vi "ClusterEscala.vi"() -> ()   [LabVIEW 2020]
panel:
  out "Cluster":T1 {"PRESION" scale=0.0..10.0; "FLUJO" scale=0.0..10.0; "TEMPERATURA" scale=0.0..100.0}
  in  "Cluster 2":T2
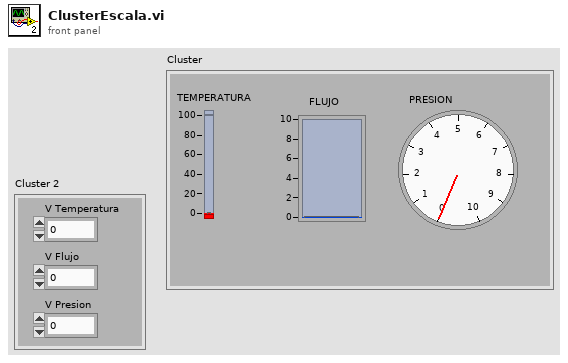
[diagram p1: front panel]
types:
  T1 = cluster{"TEMPERATURA":dbl, "FLUJO":dbl, "PRESION":dbl}
  T2 = cluster{"V Temperatura":dbl, "V Flujo ":dbl, "V Presion ":dbl}
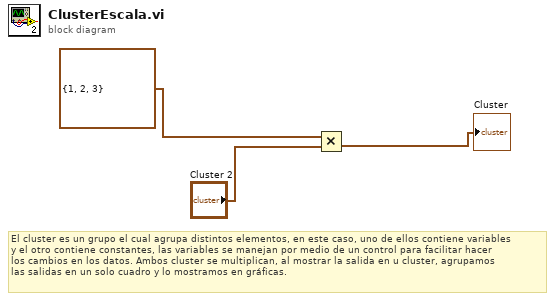
[diagram p0: block diagram]
diagram:
  # "El cluster es un grupo el cual agrupa distintos elementos, en este caso, uno de ellos contiene variables\ny el otro contiene constantes, las variables se manejan por medio de un control para facilitar hacer\nlos cambios en los datos. Ambos cluster se multiplican, al mostrar la salida en u cluster, agrupamos\nlas salidas en un solo cuadro y lo mostramos en gráficas."
  n1 = Multiply(x=cluster{i32, i32, i32} {1, 2, 3} ("Cluster"), y="Cluster 2") -> (x*y=→"Cluster":cluster{dbl, dbl, dbl})
